vi "Main_steam_Min_P_SP_correction.vi"(0 "MD420.lvclass in":refnum<class "MD420.lvclass">, 1 "Min-P Corr OFF":bool, 2 "ACT SP Ctrl OFF":bool, 3 "PUMA 1/4":bool, 4 "PR":dbl, 5 "ACT effective Setpoint":dbl, 6 "ACT upper limit":dbl, 7 "error in":errorcluster, 8 "ACT limit Setpoint":dbl, 9 "ACT lower limit":dbl) -> (20 "MD420.lvclass out":refnum<class "MD420.lvclass">, 23 "MS Min SP Corr":dbl, 27 "error out":errorcluster)   [LabVIEW 2022 SP3, in "MD420.lvclass"]
uses:
  MD420.lvclass
  MD420.lvclass/MD420.ctl
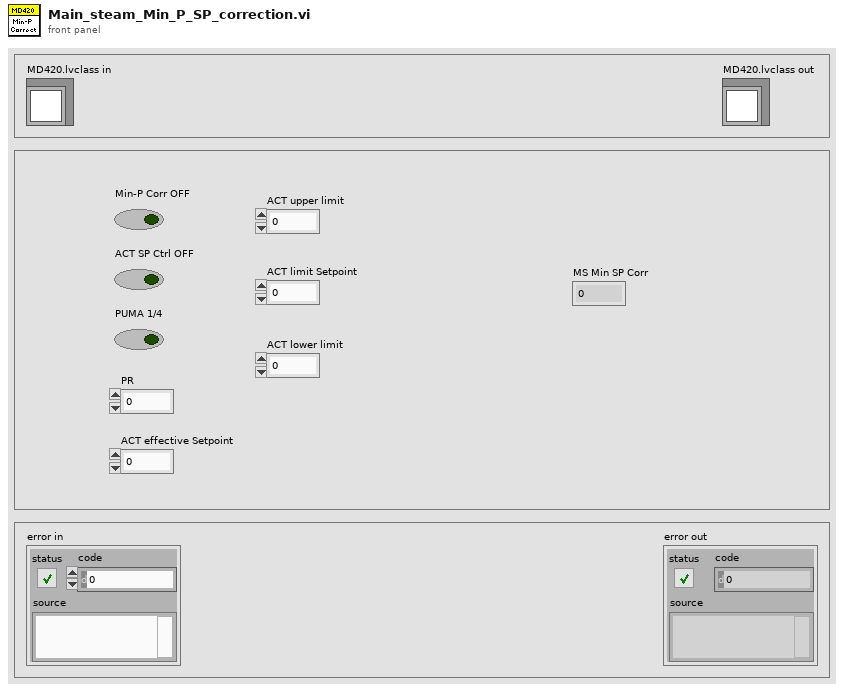
[diagram p1: front panel]
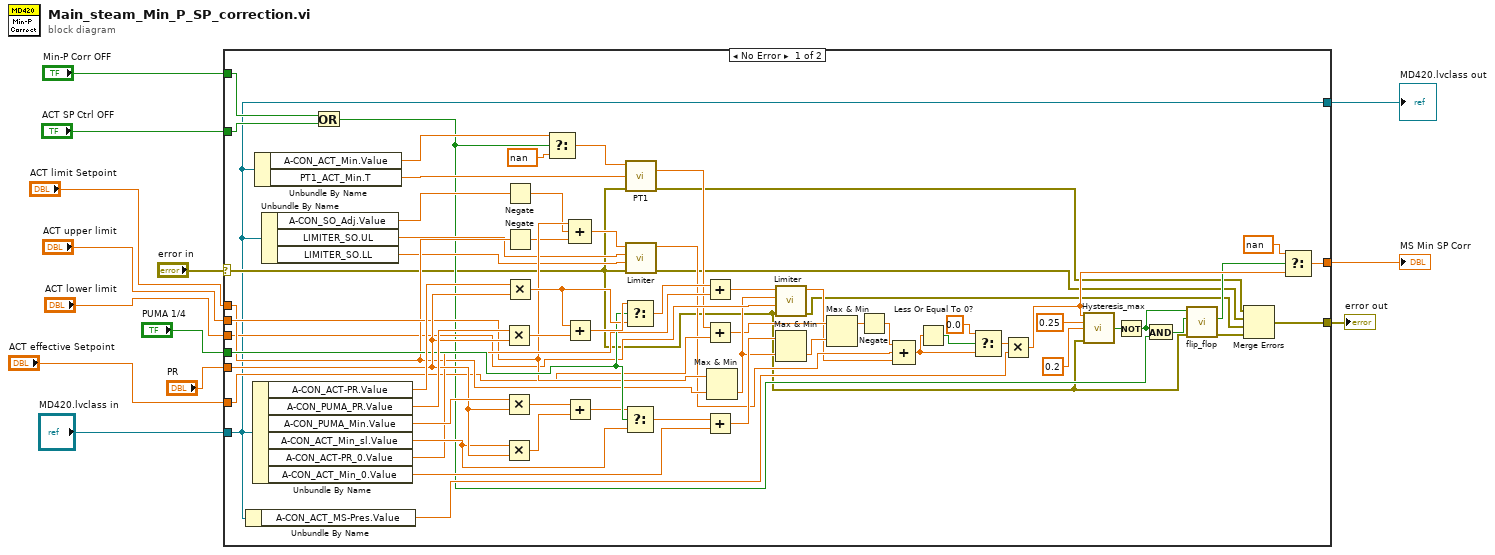
[diagram p0: block diagram]
diagram:
  n1 = case shown="No Error" "error in" {
    selector: "error in" -> [w23 w79]
    tunnel: "MD420.lvclass in" -> [w14 w78]
    tunnel: "PR" -> [w71 _]
    tunnel: "PUMA 1/4" -> [w68 _]
    tunnel: "Min-P Corr OFF" -> [w65 _]
    tunnel: "ACT SP Ctrl OFF" -> [w64 _]
    tunnel: "ACT upper limit" -> [w53 _]
    tunnel: "ACT limit Setpoint" -> [w51 _]
    tunnel: "ACT lower limit" -> [w46 _]
    tunnel: "ACT effective Setpoint" -> [w44 _]
    tunnel: [w20 _] -> w3
    tunnel: [w15 w79] -> w2
    tunnel: [w14 w78] -> w1
    frame No Error {
      n2 = Unbundle By Name(w14) -> ("A-CON_ACT_MS-Pres.Value"=w31:dbl)
      n3 = Unbundle By Name(w14) -> ("A-CON_ACT-PR.Value"=w77:dbl, "A-CON_PUMA_PR.Value"=w76:dbl, "A-CON_PUMA_Min.Value"=w72:dbl, "A-CON_ACT_Min_sl.Value"=w66:dbl, "A-CON_ACT-PR_0.Value"=w59:dbl, "A-CON_ACT_Min_0.Value"=w56:dbl)
      n4 = Unbundle By Name(w14) -> ("A-CON_ACT_Min.Value"=w63:dbl, "PT1_ACT_Min.T"=w60:dbl)
      n5 = Unbundle By Name(w14) -> ("A-CON_SO_Adj.Value"=w54:dbl, "LIMITER_SO.UL"=w48:dbl, "LIMITER_SO.LL"=w47:dbl)
      n6 = Or(x=w65, y=w64) -> (x .or. y?=w25:bool)
      n7 = Multiply(x=w76, y=w71) -> (x*y=w75:dbl)
      n8 = Multiply(x=w72, y=w71) -> (x*y=w70:dbl)
      n9 = Multiply(x=w66, y=w71) -> (x*y=w69:dbl)
      n10 = Negate(x=w54) -> (-x=w52:dbl)
      n11 = Negate(x=w51) -> (-x=w50:dbl)
      n12 = Multiply(x=w77, y=w71) -> (x*y=w73:dbl)
      n13 = Select(t=w63, s=w25, f=nan) -> (s? t:f=w61:dbl)
      n14 = Add(x=w73, y=w75) -> (x+y=w74:dbl)
      n15 = Add(x=w70, y=w69) -> (x+y=w67:dbl)
      n16 = Compound Arithmetic op=ADD(w53, w52, w50) -> (w49:dbl)
      n17 = Select(t=w74, s=w68, f=w73) -> (s? t:f=w58:dbl)
      n18 = Select(t=w67, s=w68, f=w66) -> (s? t:f=w57:dbl)
      n19 = call "PT1.vi"("input u(k)"=w61, "T1"=w60, "error in (no error)"=w23) -> ("output y(k)"=w45:dbl, "error out"=w19:errorcluster)  [unwired: 11 in]
      n20 = call "Limiter.vi"("error in"=w23, "LIMITER_PG_lift-up.LL"=w47, "LIMITER_PG_lift-up.UL in"=w48, "input"=w49) -> ("error IO"=w18:errorcluster, "LIMITER_PG_lift-up.UL out"=w37:dbl)  [unwired: 4 in, 2 out]
      n21 = Add(x=w58, y=w59) -> (x+y=w55:dbl)
      n22 = Add(x=w45, y=w44) -> (x+y=w40:dbl)
      n23 = Add(x=w57, y=w56) -> (x+y=w43:dbl)
      n24 = Max & Min(x=w53, y=w51) -> (min(x,y)=w42:dbl)  [unwired: 1 out]
      n25 = call "Limiter.vi"("error in"=w23, "LIMITER_PG_lift-up.LL"=w46, "LIMITER_PG_lift-up.UL in"=w42, "input"=w55) -> ("error IO"=w17:errorcluster, "LIMITER_PG_lift-up.UL out"=w36:dbl)  [unwired: 4 in, 2 out]
      n26 = Max & Min(x=w43, y=w42) -> (min(x,y)=w41:dbl)  [unwired: 1 out]
      n27 = Max & Min(x=w40, y=w41) -> (max(x,y)=w39:dbl)  [unwired: 1 out]
      n28 = Negate(x=w39) -> (-x=w38:dbl)
      n29 = Compound Arithmetic op=ADD(w38, w37, w36) -> (w34:dbl)
      n30 = Less Or Equal To 0?(x=w34) -> (x <= 0?=w35:bool)
      n31 = Select(t=0.0, s=w35, f=w34) -> (s? t:f=w32:dbl)
      n32 = Multiply(x=w32, y=w31) -> (x*y=w30:dbl)
      n33 = call "Hysteresis_max.vi"("input(+)"=w30, "input (-)"=0.25, "H"=0.2, "error in"=w23) -> ("Deviation"=w27:bool)  [unwired: 10 in, 1 out]
      n34 = Not(x=w27) -> (.not. x?=w26:bool)
      n35 = And(x=w26, y=w25) -> (x .and. y?=w24:bool)
      n36 = call "flip_flop.vi"("error in"=w23, "BI2"=w24, "BI1"=w26) -> ("error out"=w16:errorcluster, "BO2"=w22:bool)  [unwired: 6 in, 1 out]
      n37 = Merge Errors(w19, w18, w17, w16) -> (w15:errorcluster)
      n38 = Select(t=nan, s=w22, f=w30) -> (s? t:f=w20:dbl)
    }
    frame Error {
    }
  }
  "MS Min SP Corr" <- w3
  "error out" <- w2
  "MD420.lvclass out" <- w1
